vi "ALTS-2015 Read Scan Data.vi"(8 "error in (no error)":errorcluster, 9 "timeout ms":i32=1000, 11 "connection ID":refnum<k5>) -> (0 "error out":errorcluster, 2 "data out":string, 3 "connection ID out":refnum<k5>)   [LabVIEW 2013]
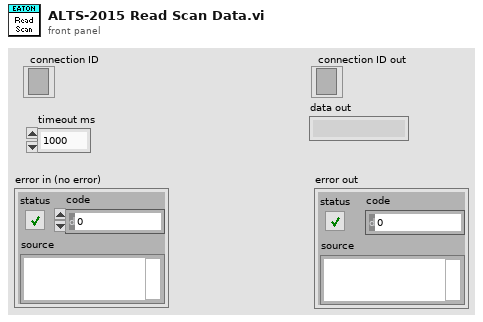
[diagram p1: front panel]
types:
  T1 = enum16{"Standard", "Buffered", "CRLF", "Immediate"}
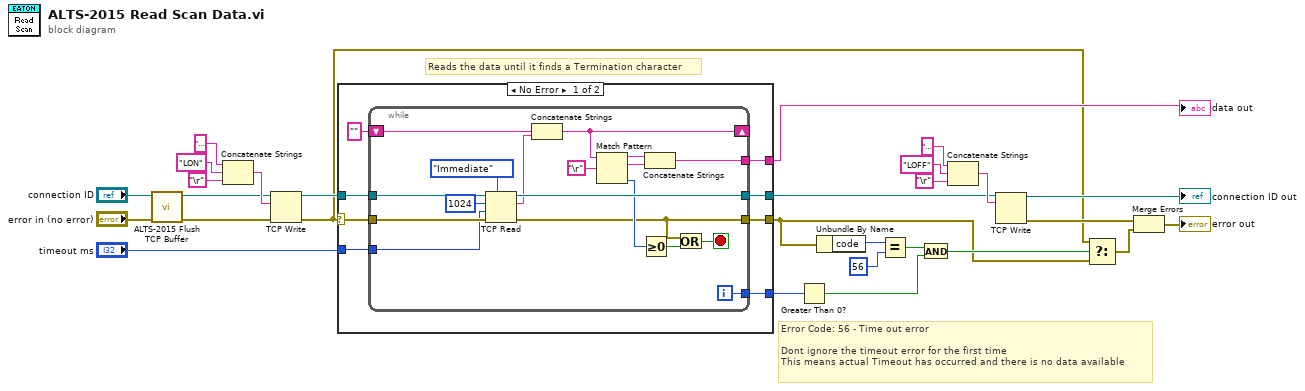
[diagram p0: block diagram]
diagram:
  # "Error Code: 56 - Time out error\n\nDont ignore the timeout error for the first time\nThis means actual Timeout has occurred and there is no data available"
  # "Reads the data until it finds a Termination character"
  n1 = call "ALTS-2015 Flush TCP Buffer.vi"("error in (no error)"="error in (no error)", "TCP Connection in"="connection ID") -> ("error out"=w13:errorcluster, "TCP Connection out"=w14:refnum<k5>)  [unwired: 8 in]
  n2 = Concatenate Strings("\u001b", "LON", "\r" ("string")) -> (w27:string)
  n3 = TCP Write(connection ID=w14, data in=w27, error in (no error)=w13) -> (connection ID out=w26:refnum<k5>, error out=w1:errorcluster)  [unwired: 2 out]
  n4 = case shown="No Error" w1 {
    selector: w1 -> [w33 w55]
    tunnel: w26 -> [w36 w56]
    tunnel: [w35 w56] -> w19
    tunnel: [w34 w55] -> w3
    tunnel: "timeout ms" -> [w32 _]
    tunnel: [w30 _] -> w7
    tunnel: [w29 _] -> w2
    frame No Error {
      n5 = while {
        tunnel: w36 -> [w53]
        tunnel: w33 -> [w52]
        tunnel: [w51] -> w35
        tunnel: [w38] -> w34
        tunnel: w32 -> [w50]
        shift-right: [w42] -> _
        shift-left: "" -> [w47]
        tunnel: [w46] -> w30
        tunnel: [w37] -> w29
        i -> [w46]
        stop <- w41 stop-if-true
        n6 = TCP Read(connection ID=w53, bytes to read=1024, error in (no error)=w52, 7:T1."Immediate" ("mode (standard)"), 9:w50) -> (connection ID out=w51:refnum<k5>, data out=w48:string, error out=w38:errorcluster)
        n7 = Concatenate Strings(w47, w48) -> (w42:string)
        n8 = Match Pattern(string=w42, regular expression="\r" ("string")) -> (before substring=w44:string, match substring=w45:string, offset past match=w39:i32)  [unwired: 1 in, 1 out]
        n9 = Greater Or Equal To 0?(x=w39) -> (x >= 0?=w40:bool)
        n10 = Concatenate Strings(w44, w45) -> (w37:string)
        n11 = Or(x=w38, y=w40) -> (x .or. y?=w41:bool)
      }
    }
    frame Error {
    }
  }
  "data out" <- w2
  n12 = Greater Than 0?(x=w7) -> (x > 0?=w6:bool)
  n13 = Unbundle By Name(w3) -> ("code"=w9:i32)
  n14 = Equal?(x=w9, y=56) -> (x = y?=w5:bool)
  n15 = And(x=w5, y=w6) -> (x .and. y?=w4:bool)
  n16 = Concatenate Strings("\u001b", "LOFF", "\r" ("string")) -> (w22:string)
  n17 = TCP Write(connection ID=w19, data in=w22) -> (connection ID out=→"connection ID out":refnum<k5>, error out=w18:errorcluster)  [unwired: 1 in, 2 out]
  n18 = Select(t=w1, s=w4, f=w3) -> (s? t:f=w8:errorcluster)
  n19 = Merge Errors(w18, w8) -> (→"error out":errorcluster)
